vi "Lakeshore218Parse.vi"(11 "Resistance String":string) -> (2 "Low Level (Ohms)":dbl, 3 "High Level (Ohms)":dbl)   [LabVIEW 2018]
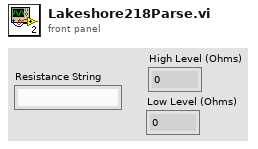
[diagram p1: front panel]
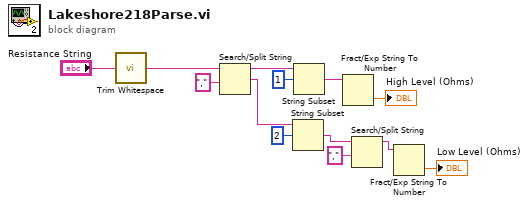
[diagram p0: block diagram]
diagram:
  n1 = call "Trim Whitespace.vi"("string"="Resistance String") -> ("trimmed string"=w12:string)  [unwired: 1 in]
  n2 = Search/Split String(string=w12, search string/char (-)=",") -> (substring before match=w9:string, match + rest of string=w5:string)  [unwired: 1 in, 1 out]
  n3 = String Subset(string=w5, offset (0)=2) -> (substring=w3:string)  [unwired: 1 in]
  n4 = String Subset(string=w9, offset (0)=1) -> (substring=w8:string)  [unwired: 1 in]
  n5 = Fract/Exp String To Number(string=w8) -> (number=→"High Level (Ohms)":dbl)  [unwired: 3 in, 1 out]
  n6 = Search/Split String(string=w3, search string/char (-)=",") -> (substring before match=w1:string)  [unwired: 1 in, 2 out]
  n7 = Fract/Exp String To Number(string=w1) -> (number=→"Low Level (Ohms)":dbl)  [unwired: 3 in, 1 out]
